vi "Autonomous Independent.vi"() -> ()   [LabVIEW 2015]
doc: "This VI is called when autonomous begins, and will automatically be terminated when autonomous ends. You can carry out timed or sensor driven robot movement independently without needing to return to the caller."
uses:
  <vilib>/Rock Robotics/WPI/Utilities/WPI_GetSetVariantRefNum.vi
  <vilib>/Rock Robotics/Network Tables/NT Read Number.vi
  Robot Global Data.vi
  <vilib>/Rock Robotics/WPI/RobotDrive/WPI_RobotDriveMecanumDrive_Cartesian.vi
  <vilib>/Rock Robotics/Network Tables/NT Write Numeric Array.vi
  <vilib>/Rock Robotics/Network Tables/NT Read Boolean.vi
panel:
  out "Drive Time":dbl
  # "Be sure to right-click and choose Data Operations>>Make Current Value default if you want to save the array values with the VI"
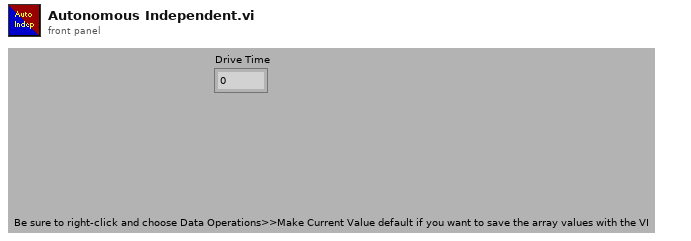
[diagram p1: front panel]
types:
  T1 = typedef "WPI_JoystickDevRef.ctl" = cluster{"Device":T2}
  T2 = typedef "WPI_JoystickDeviceEnum.ctl" = enum16{"USB 0", "USB 1", "USB 2", "USB 3", "USB 4", "USB 5"}
  T3 = typedef "WPI_AccelerometerDevRef.ctl" = cluster{"DevStatus":errorcluster, "Scaling":T4, "Analog Channels":T5, "I2C Bus":T7, "SPI Bus":T8, "Accel Range":T9, "ADXL Axes":T10, "Handle":i32, "Device Address":u8, "Accel Type":enum16{"Analog", "ADXL345 I2C", "ADXL345 SPI", "Internal", "ADXL362 SPI"}}
  T4 = typedef "WPI_AccelerometerScaling.ctl" = cluster{"Gain (VoltsPerG)":dbl, "Center Voltage":dbl}
  T5 = typedef "WPI_AccelerometerAnalogChannels.ctl" = cluster{"X-Axis":T6, "Y-Axis":T6, "Z-Axis":T6}
  T6 = typedef "FPGA_AIChannel.ctl" = enum8{"AI 0", "AI 1", "AI 2", "AI 3", "AI MXP 0", "AI MXP 1", "AI MXP 2", "AI MXP 3", "Invalid"}
  T7 = typedef "i2c_bus.ctl" = enum16{"I2C On-Board", "I2C MXP", "Invalid"}
  T8 = typedef "spi_bus.ctl" = enum16{"SPI On-Board, CS0", "SPI On-Board, CS1", "SPI On-Board, CS2", "SPI On-Board, CS3", "SPI MXP", "Invalid"}
  T9 = typedef "ADXL345 Range.ctl" = u8
  T10 = typedef "WPI_AccelerometerADXL345 Axes.ctl" = cluster{"X-Axis":bool, "Y-Axis":bool, "Z-Axis":bool}
  T11 = typedef "WPI_MotorControlDeviceRef.ctl" = cluster{"DeviceStatus":errorcluster, "Type":T12, "PWM":cluster{"PWM Channel":T13, "DeadBand":T14}, "CAN":cluster{"Device Number":u8, "Control Mode":T15, "Semaphore":T16, "Max Vout":dbl, "TalonSRX Control Mode":T17}, "Invert":bool}
  T12 = typedef "WPI_MotorControlType.ctl" = enum16{"PWM", "CAN", "CANTalonSRX"}
  T13 = typedef "FPGA_DIOPWMChannel.ctl" = enum8{"PWM 0", "PWM 1", "PWM 2", "PWM 3", "PWM 4", "PWM 5", "PWM 6", "PWM 7", "PWM 8", "PWM 9", "PWM MXP 0", "PWM MXP 1", "PWM MXP 2", "PWM MXP 3", "PWM MXP 4", "PWM MXP 5", "PWM MXP 6", "PWM MXP 7", "PWM MXP 8", "PWM MXP 9", "Invalid"}
  T14 = typedef "WPI_PWMDeadband.ctl" = cluster{"Name":string, "maxPositivePwm":i32, "minPositivePwm":i32, "centerPwm":i32, "maxNegativePwm":i32, "minNegativePwm":i32, "angularRange":u16}
  T15 = typedef "WPI_CANJaguar_ControlMode.ctl" = enum8{"Percent VBus", "Current", "Speed", "Position", "Voltage"}
  T16 = typedef "Semaphore RefNum" = refnum<k1>
  T17 = typedef "WPI_CANTalonSRX_APIControlMode.ctl" = enum8{"Percent VBus", "Speed", "Position", "Slave", "Unchanged / Invalid", "Voltage Compensation", "Current", "Motion Profile"}
  T18 = typedef "WPI_RobotDriveDevRef.ctl" = cluster{"DevStatus":errorcluster, "Motors[]":T11[], "Square Inputs":bool, "Max Output":dbl}
  T19 = typedef "eventsource.ctl" = u32
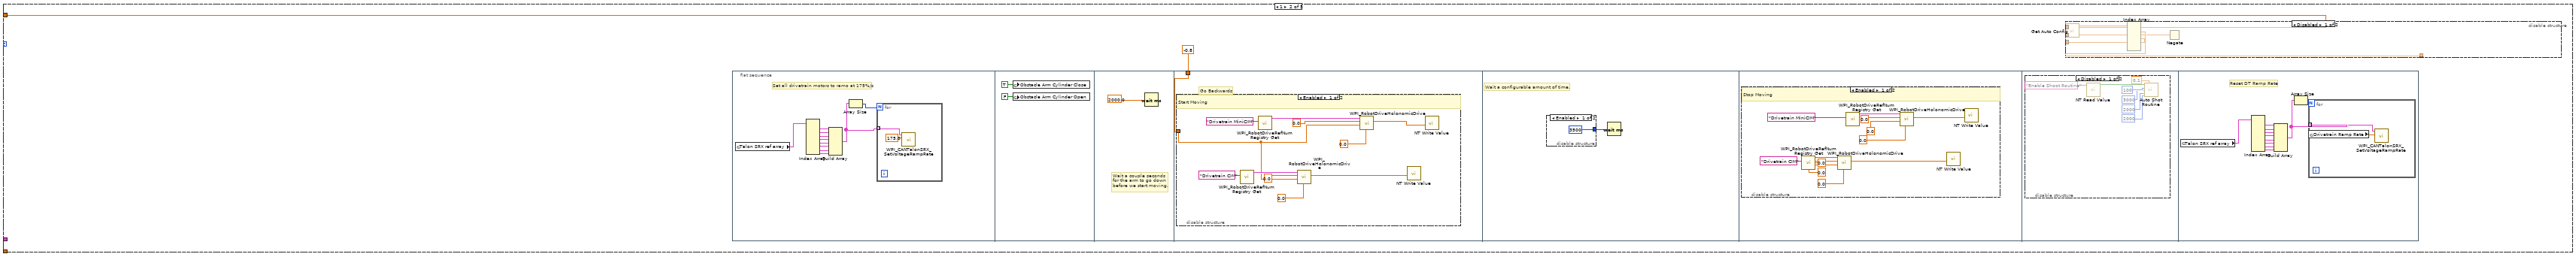
[diagram p3: hidden frame]
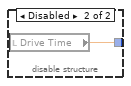
[diagram p6: hidden frame]
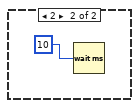
[diagram p14: hidden frame]
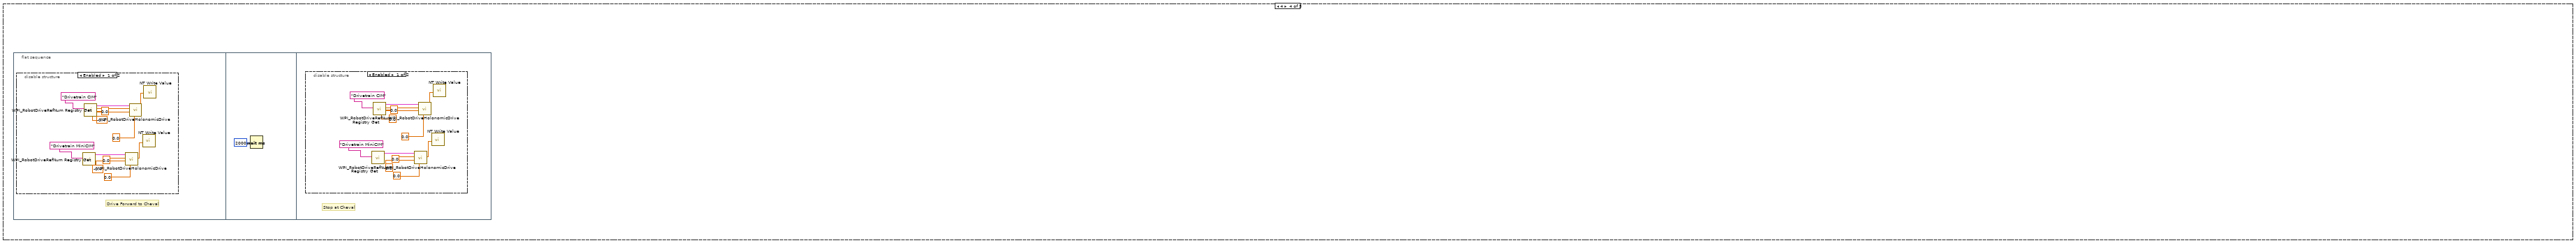
[diagram p19: hidden frame]
diagram:
  (unwired) "This function is run in parallel when the autonomous period begins. It will be terminated automatically when the period ends.\n\nNote that all Driver Station inputs are automatically latched and will not change once auto begins."
  # "Low Bar/Portcullis Auto Routine, with optional shoot routine."
  # "This tells you the autonomous selected\nfrom the dashboard"
  # "Every 20ms, report that we are running autonomous\ncode. Loop will abort the same time as the VI."
  # "This gives you the joystick value\nthat is often the throttle"
  # "This tells you the driver position\nand alliance color"
  n1 = while {
    stop <- FALSE stop-if-true
    n2 = call <vilib>:"WPI_DriverStationReport Robot Code State.vi"("Autonomous"=TRUE) -> ()  [unwired: 10 in, 1 out]
    n3 = Wait (ms)(milliseconds to wait=u32 20) -> ()  [unwired: 1 out]
  }
  n4 = call <vilib>:"WPI_DriverStationGet Alliance Info.vi"() -> ()  [unwired: 12 out]
  n5 = call <vilib>:"WPI_JoystickRefNum Registry Get.vi"("refnum name"="Joystick 0") -> ("JoystickDevRef"=w10:T1)  [unwired: 1 in, 9 out]
  n6 = disable-structure shown="Enabled" {
    disable-tunnel: [w16 _] -> w4
    frame Enabled {
      n7 = call-poly <vilib>:"NT Read Value.vi"("Name"="Drive Time") -> ("Numeric"=w16:dbl)  [unwired: 9 in, 1 out]
    }
    frame Disabled {
    }
  }
  n8 = call <vilib>:"WPI_JoystickGetValues.vi"("JoystickDevRef"=w10) -> ("Axes"=w7:dbl[])  [unwired: 6 in, 4 out]
  n9 = call-poly <vilib>:"NT Read Value.vi"("Name"="Select Autonomous") -> ("Numeric"=w5:dbl)  [unwired: 9 in, 1 out]
  n10 = local write "Drive Time"(w4) -> ()
  n11 = call-poly <vilib>:"NT Write Value.vi"("Numeric Array"=w7, "Name"="Joystick 0/Axes") -> ()  [unwired: 9 in, 1 out]
  n12 = Index Array(array=w7, index=2) -> ()  [unwired: 1 out]
  n13 = flat-sequence {
    tunnel: w5 -> [w20]
    tunnel: [w20] -> w3
    tunnel: [w18] -> w2
    tunnel: [w17] -> w1
    tunnel: w3 -> [w23]
    tunnel: w2 -> [w22]
    tunnel: w1 -> [w21]
    frame #0 {
      # "Initialize Accel."
      n14 = call "2039_GetAccelDeltas.vi"("refnum name"="Internal Accel") -> ("Deltas to apply"=w17:dbl[], "AccelerometerDevRef"=w18:T3)  [unwired: 2 in, 1 out]
    }
    frame #1 {
      n15 = case shown="3" w23 {
        tunnel: w23 -> [_ w25 _ _ _]
        tunnel: w22 -> [_ _ w100 _ _]
        tunnel: w21 -> [_ _ w99 _ _]
        frame 0, Default {
        }
        frame 1 {
          n16 = flat-sequence {
            tunnel: -0.8 -> [w48]
            frame #0 {
              # "Set all drivetrain motors to ramo at 175%/s"
              n17 = global read "Robot Global Data.vi" "Talon SRX ref array"() -> (w42:T11[])
              n18 = Index Array(array=w42) -> (element #1=w35:T11, element #2=w34:T11, element #3=w36:T11, element #4=w37:T11, element #5=w38:T11, element #6=w39:T11, element #7=w40:T11, element #8=w41:T11)  [unwired: 8 in]
              n19 = Build Array(w35, w34, w36, w37, w38, w39, w40, w41) -> (w32:T11[])
              n20 = Array Size(array=w32) -> (size(s)=w33:i32)
              n21 = for {
                N: w33 -> [_]
                tunnel: w32 -> [w44] mode=indexing
                n22 = call <vilib>:"WPI_CANTalonSRX_SetVoltageRampRate.vi"("Throttle Ramp Rate (percent/s)"=175.0, "CAN Talon SRX Ref"=w44) -> ()  [unwired: 8 in, 2 out]
              }
            }
            frame #1 {
              n23 = global write "Robot Global Data.vi" "Obstacle Arm Cylinder Close"(TRUE) -> ()
              n24 = global write "Robot Global Data.vi" "Obstacle Arm Cylinder Open"(FALSE) -> ()
            }
            frame #2 {
              # "Wait a couple seconds\nfor the arm to go down\nbefore we start moving."
              n25 = Wait (ms)(milliseconds to wait=2000.0) -> ()  [unwired: 1 out]
            }
            frame #3 {
              # "Go Backwards"
              n26 = disable-structure shown="Enabled" {
                disable-tunnel: w48 -> [w50 _]
                frame Enabled {
                  # "Start Moving"
                  n27 = call <vilib>:"WPI_RobotDriveRefNum Registry Get.vi"("refnum name"="Drivetrain CIM") -> ("RobotDriveDevRef"=w56:T18)  [unwired: 1 in, 9 out]
                  n28 = call <vilib>:"WPI_RobotDriveRefNum Registry Get.vi"("refnum name"="Drivetrain MiniCIM") -> ("RobotDriveDevRef"=w52:T18)  [unwired: 1 in, 9 out]
                  n29 = call-poly <vilib>:"WPI_RobotDriveHolonomicDrive.vi"("Rotation"=0.0, "Y"=w50, "X"=0.0 ("X axis value"), "RobotDriveDevRef"=w56) -> ("Motor Values"=w57:dbl[])  [unwired: 5 in, 2 out]
                  n30 = call-poly <vilib>:"WPI_RobotDriveHolonomicDrive.vi"("Rotation"=0.0, "Y"=w50, "X"=0.0 ("X axis value"), "RobotDriveDevRef"=w52) -> ("Motor Values"=w54:dbl[])  [unwired: 5 in, 2 out]
                  n31 = call-poly <vilib>:"NT Write Value.vi"("Numeric Array"=w57) -> ()  [unwired: 10 in, 1 out]
                  n32 = call-poly <vilib>:"NT Write Value.vi"("Numeric Array"=w54) -> ()  [unwired: 10 in, 1 out]
                }
                frame Disabled {
                }
              }
            }
            frame #4 {
              # "Wait a configurable amount of time."
              n33 = disable-structure shown="Enabled" {
                disable-tunnel: [u32 3500 ("milliseconds to wait") w62] -> w60
                frame Enabled {
                }
                frame Disabled {
                  n34 = local read "Drive Time"() -> (w62:dbl)
                }
              }
              n35 = Wait (ms)(milliseconds to wait=w60) -> ()  [unwired: 1 out]
            }
            frame #5 {
              n36 = disable-structure shown="Enabled" {
                frame Enabled {
                  # "Stop Moving"
                  n37 = call <vilib>:"WPI_RobotDriveRefNum Registry Get.vi"("refnum name"="Drivetrain CIM") -> ("RobotDriveDevRef"=w70:T18)  [unwired: 1 in, 9 out]
                  n38 = call-poly <vilib>:"WPI_RobotDriveHolonomicDrive.vi"("Rotation"=0.0, "Y"=0.0 ("X axis value"), "X"=0.0 ("X axis value"), "RobotDriveDevRef"=w70) -> ("Motor Values"=w71:dbl[])  [unwired: 5 in, 2 out]
                  n39 = call <vilib>:"WPI_RobotDriveRefNum Registry Get.vi"("refnum name"="Drivetrain MiniCIM") -> ("RobotDriveDevRef"=w64:T18)  [unwired: 1 in, 9 out]
                  n40 = call-poly <vilib>:"WPI_RobotDriveHolonomicDrive.vi"("Rotation"=0.0, "Y"=0.0 ("X axis value"), "X"=0.0 ("X axis value"), "RobotDriveDevRef"=w64) -> ("Motor Values"=w66:dbl[])  [unwired: 5 in, 2 out]
                  n41 = call-poly <vilib>:"NT Write Value.vi"("Numeric Array"=w71) -> ()  [unwired: 10 in, 1 out]
                  n42 = call-poly <vilib>:"NT Write Value.vi"("Numeric Array"=w66) -> ()  [unwired: 10 in, 1 out]
                }
                frame Disabled {
                }
              }
            }
            frame #6 {
              n43 = disable-structure shown="Disabled" {
                frame Disabled {
                  n44 = call-poly <vilib>:"NT Read Value.vi"("Name"="Enable Shoot Routine") -> ("Boolean"=w80:bool)  [unwired: 9 in, 1 out]
                  n45 = call "Auto Shot Routine.vi"("Enable"=w80, "Speed to run intake motor (negated)"=0.1, "Time to wait after boulder out"=100, 7:3000, "Wait for SpinUp"=2000, "Wait for Shot Time"=2000) -> ()  [unwired: 10 in]
                }
                frame Enabled {
                }
              }
            }
            frame #7 {
              # "Reset DT Ramp Rate"
              n46 = global read "Robot Global Data.vi" "Talon SRX ref array"() -> (w92:T11[])
              n47 = Index Array(array=w92) -> (element #1=w85:T11, element #2=w84:T11, element #3=w86:T11, element #4=w87:T11, element #5=w88:T11, element #6=w89:T11, element #7=w90:T11, element #8=w91:T11)  [unwired: 8 in]
              n48 = Build Array(w85, w84, w86, w87, w88, w89, w90, w91) -> (w82:T11[])
              n49 = Array Size(array=w82) -> (size(s)=w83:i32)
              n50 = for {
                N: w83 -> [_]
                tunnel: w82 -> [w94] mode=indexing
                n51 = global read "Robot Global Data.vi" "Drivetrain Ramp Rate"() -> (w93:dbl)
                n52 = call <vilib>:"WPI_CANTalonSRX_SetVoltageRampRate.vi"("Throttle Ramp Rate (percent/s)"=w93, "CAN Talon SRX Ref"=w94) -> ()  [unwired: 8 in, 2 out]
              }
            }
          }
          n53 = disable-structure shown="Disabled" {
            disable-tunnel: w25 -> [w30 _]
            disable-tunnel: [w29 _] -> _
            disable-tunnel: [w27 _] -> _
            disable-tunnel: [w26 _] -> _
            frame Disabled {
              n54 = call "Get Auto Config.vi"("Numeric"=w30) -> ("Numeric Array"=w31:dbl[])  [unwired: 10 in]
              n55 = Index Array(array=w31) -> (element #1=w29:dbl, element #2=w28:dbl, element #3=w26:dbl)  [unwired: 6 in, 3 out]
              n56 = Negate(x=w28) -> (-x=w27:dbl)
            }
            frame Enabled {
            }
          }
        }
        frame 2 {
          # "Hopefully this will run in parallel"
          # "Can be written as needed..."
          n57 = flat-sequence {
            tunnel: w97 -> [w113]
            tunnel: [w111] -> _
            tunnel: [w111] -> w96
            tunnel: w96 -> [w116]
            tunnel: [w116] -> w95
            tunnel: w95 -> [w125]
            frame #0 {
              n58 = disable-structure shown="Enabled" {
                frame Enabled {
                  w101 = 0.0
                  w102 = 0.0 ("X axis value")
                  # "Start Moving"
                  n59 = call <vilib>:"WPI_RobotDriveRefNum Registry Get.vi"("refnum name"="Drivetrain CIM") -> ("RobotDriveDevRef"=w108:T18)  [unwired: 1 in, 9 out]
                  n60 = call <vilib>:"WPI_RobotDriveRefNum Registry Get.vi"("refnum name"="Drivetrain MiniCIM") -> ("RobotDriveDevRef"=w105:T18)  [unwired: 1 in, 9 out]
                  n61 = call-poly <vilib>:"WPI_RobotDriveHolonomicDrive.vi"("Rotation"=w102, "Y"=-0.8 ("X axis value"), "X"=w102, "RobotDriveDevRef"=w105) -> ("Motor Values"=w107:dbl[])  [unwired: 5 in, 2 out]
                  n62 = call-poly <vilib>:"WPI_RobotDriveHolonomicDrive.vi"("Rotation"=w101, "Y"=-0.8, "X"=w101, "RobotDriveDevRef"=w108) -> ("Motor Values"=w109:dbl[])  [unwired: 5 in, 2 out]
                  n63 = call-poly <vilib>:"NT Write Value.vi"("Numeric Array"=w109) -> ()  [unwired: 10 in, 1 out]
                  n64 = call-poly <vilib>:"NT Write Value.vi"("Numeric Array"=w107) -> ()  [unwired: 10 in, 1 out]
                }
                frame Disabled {
                }
              }
            }
            frame #1 {
              n65 = event shown="[0] <Acceleration Spike Event>: User Event;  Timeout" {
                selector: w113 -> [_]
                dyn-events: _ -> [_]
                timeout: 2500 -> [_]
                tunnel: [w114] -> w111
                event User Event; Timeout {
                  # "Wait until either Timeout or accel change."
                  n66 = event-data() -> ("Source"=w114:T19)  [unwired: 1 in, 2 out]
                  n67 = Wait (ms)(milliseconds to wait=10) -> ()  [unwired: 1 out]
                }
              }
            }
            frame #2 {
              n68 = disable-structure shown="Enabled" {
                frame Enabled {
                  w117 = 0.0
                  w118 = 0.0 ("X axis value")
                  # "Stop Moving"
                  n69 = call <vilib>:"WPI_RobotDriveRefNum Registry Get.vi"("refnum name"="Drivetrain CIM") -> ("RobotDriveDevRef"=w122:T18)  [unwired: 1 in, 9 out]
                  n70 = call <vilib>:"WPI_RobotDriveRefNum Registry Get.vi"("refnum name"="Drivetrain MiniCIM") -> ("RobotDriveDevRef"=w119:T18)  [unwired: 1 in, 9 out]
                  n71 = call-poly <vilib>:"WPI_RobotDriveHolonomicDrive.vi"("Rotation"=w117, "Y"=w117, "X"=w117, "RobotDriveDevRef"=w122) -> ("Motor Values"=w123:dbl[])  [unwired: 5 in, 2 out]
                  n72 = call-poly <vilib>:"WPI_RobotDriveHolonomicDrive.vi"("Rotation"=w118, "Y"=w118, "X"=w118, "RobotDriveDevRef"=w119) -> ("Motor Values"=w121:dbl[])  [unwired: 5 in, 2 out]
                  n73 = call-poly <vilib>:"NT Write Value.vi"("Numeric Array"=w123) -> ()  [unwired: 10 in, 1 out]
                  n74 = call-poly <vilib>:"NT Write Value.vi"("Numeric Array"=w121) -> ()  [unwired: 10 in, 1 out]
                }
                frame Disabled {
                }
              }
            }
            frame #3 {
              n75 = case shown="1, Default" w125 {
                frame 1, Default {
                  # "Back up a smidge if we timed out"
                  n76 = flat-sequence {
                    frame #0 {
                      n77 = disable-structure shown="Enabled" {
                        frame Enabled {
                          n78 = call <vilib>:"WPI_RobotDriveRefNum Registry Get.vi"("refnum name"="Drivetrain CIM") -> ("RobotDriveDevRef"=w133:T18)  [unwired: 1 in, 9 out]
                          n79 = call <vilib>:"WPI_RobotDriveRefNum Registry Get.vi"("refnum name"="Drivetrain MiniCIM") -> ("RobotDriveDevRef"=w127:T18)  [unwired: 1 in, 9 out]
                          n80 = call-poly <vilib>:"WPI_RobotDriveHolonomicDrive.vi"("Rotation"=0.0, "Y"=0.0 ("X axis value"), "X"=0.5 ("X axis value"), "RobotDriveDevRef"=w127) -> ("Motor Values"=w128:dbl[])  [unwired: 5 in, 2 out]
                          n81 = call-poly <vilib>:"WPI_RobotDriveHolonomicDrive.vi"("Rotation"=0.0, "Y"=0.5 ("X axis value"), "X"=0.0 ("X axis value"), "RobotDriveDevRef"=w133) -> ("Motor Values"=w134:dbl[])  [unwired: 5 in, 2 out]
                          n82 = call-poly <vilib>:"NT Write Value.vi"("Numeric Array"=w128) -> ()  [unwired: 10 in, 1 out]
                          n83 = call-poly <vilib>:"NT Write Value.vi"("Numeric Array"=w134) -> ()  [unwired: 10 in, 1 out]
                        }
                        frame Disabled {
                        }
                      }
                    }
                    frame #1 {
                      n84 = Wait (ms)(milliseconds to wait=300) -> ()  [unwired: 1 out]
                    }
                    frame #2 {
                      n85 = disable-structure shown="Enabled" {
                        frame Enabled {
                          n86 = call <vilib>:"WPI_RobotDriveRefNum Registry Get.vi"("refnum name"="Drivetrain CIM") -> ("RobotDriveDevRef"=w146:T18)  [unwired: 1 in, 9 out]
                          n87 = call <vilib>:"WPI_RobotDriveRefNum Registry Get.vi"("refnum name"="Drivetrain MiniCIM") -> ("RobotDriveDevRef"=w140:T18)  [unwired: 1 in, 9 out]
                          n88 = call-poly <vilib>:"WPI_RobotDriveHolonomicDrive.vi"("Rotation"=0.0, "Y"=0.0 ("X axis value"), "X"=0.0 ("X axis value"), "RobotDriveDevRef"=w140) -> ("Motor Values"=w141:dbl[])  [unwired: 5 in, 2 out]
                          n89 = call-poly <vilib>:"WPI_RobotDriveHolonomicDrive.vi"("Rotation"=0.0, "Y"=0.0 ("X axis value"), "X"=0.0 ("X axis value"), "RobotDriveDevRef"=w146) -> ("Motor Values"=w147:dbl[])  [unwired: 5 in, 2 out]
                          n90 = call-poly <vilib>:"NT Write Value.vi"("Numeric Array"=w141) -> ()  [unwired: 10 in, 1 out]
                          n91 = call-poly <vilib>:"NT Write Value.vi"("Numeric Array"=w147) -> ()  [unwired: 10 in, 1 out]
                        }
                        frame Disabled {
                        }
                      }
                    }
                  }
                }
                frame 2 {
                  n92 = Wait (ms)(milliseconds to wait=10) -> ()  [unwired: 1 out]
                }
              }
            }
            frame #4 {
              n93 = global write "Robot Global Data.vi" "Obstacle Arm Cylinder Close"(TRUE) -> ()
              n94 = global write "Robot Global Data.vi" "Obstacle Arm Cylinder Open"(FALSE) -> ()
            }
            frame #5 {
              n95 = Wait (ms)(milliseconds to wait=2000) -> ()  [unwired: 1 out]
            }
            frame #6 {
              # "Go forth and conquer, o brave one."
              n96 = flat-sequence {
                frame #0 {
                  n97 = disable-structure shown="Enabled" {
                    frame Enabled {
                      n98 = call <vilib>:"WPI_RobotDriveRefNum Registry Get.vi"("refnum name"="Drivetrain CIM") -> ("RobotDriveDevRef"=w162:T18)  [unwired: 1 in, 9 out]
                      n99 = call <vilib>:"WPI_RobotDriveRefNum Registry Get.vi"("refnum name"="Drivetrain MiniCIM") -> ("RobotDriveDevRef"=w156:T18)  [unwired: 1 in, 9 out]
                      n100 = call-poly <vilib>:"WPI_RobotDriveHolonomicDrive.vi"("Rotation"=0.0, "Y"=0.0 ("X axis value"), "X"=-1.0 ("X axis value"), "RobotDriveDevRef"=w156) -> ("Motor Values"=w157:dbl[])  [unwired: 5 in, 2 out]
                      n101 = call-poly <vilib>:"WPI_RobotDriveHolonomicDrive.vi"("Rotation"=0.0, "Y"=-1.0 ("X axis value"), "X"=0.0 ("X axis value"), "RobotDriveDevRef"=w162) -> ("Motor Values"=w163:dbl[])  [unwired: 5 in, 2 out]
                      n102 = call-poly <vilib>:"NT Write Value.vi"("Numeric Array"=w157) -> ()  [unwired: 10 in, 1 out]
                      n103 = call-poly <vilib>:"NT Write Value.vi"("Numeric Array"=w163) -> ()  [unwired: 10 in, 1 out]
                    }
                    frame Disabled {
                    }
                  }
                }
                frame #1 {
                  n104 = Wait (ms)(milliseconds to wait=3500) -> ()  [unwired: 1 out]
                }
                frame #2 {
                  n105 = disable-structure shown="Enabled" {
                    frame Enabled {
                      n106 = call <vilib>:"WPI_RobotDriveRefNum Registry Get.vi"("refnum name"="Drivetrain CIM") -> ("RobotDriveDevRef"=w175:T18)  [unwired: 1 in, 9 out]
                      n107 = call <vilib>:"WPI_RobotDriveRefNum Registry Get.vi"("refnum name"="Drivetrain MiniCIM") -> ("RobotDriveDevRef"=w169:T18)  [unwired: 1 in, 9 out]
                      n108 = call-poly <vilib>:"WPI_RobotDriveHolonomicDrive.vi"("Rotation"=0.0, "Y"=0.0 ("X axis value"), "X"=0.0 ("X axis value"), "RobotDriveDevRef"=w169) -> ("Motor Values"=w170:dbl[])  [unwired: 5 in, 2 out]
                      n109 = call-poly <vilib>:"WPI_RobotDriveHolonomicDrive.vi"("Rotation"=0.0, "Y"=0.0 ("X axis value"), "X"=0.0 ("X axis value"), "RobotDriveDevRef"=w175) -> ("Motor Values"=w176:dbl[])  [unwired: 5 in, 2 out]
                      n110 = call-poly <vilib>:"NT Write Value.vi"("Numeric Array"=w170) -> ()  [unwired: 10 in, 1 out]
                      n111 = call-poly <vilib>:"NT Write Value.vi"("Numeric Array"=w176) -> ()  [unwired: 10 in, 1 out]
                    }
                    frame Disabled {
                    }
                  }
                }
              }
            }
          }
          n112 = call "2039_AccelSpike.vi"("Threshold"=1.0, "Delta Array"=w99, "AccelerometerDevRef"=w100) -> ("Event Registration Refnum"=w97:refnum<event-registration>)  [unwired: 7 in, 1 out]
          n113 = flat-sequence {
            frame #0 {
              n114 = disable-structure shown="Enabled" {
                frame Enabled {
                  n115 = call <vilib>:"WPI_RobotDriveRefNum Registry Get.vi"("refnum name"="Drivetrain MiniCIM") -> ("RobotDriveDevRef"=w181:T18)  [unwired: 1 in, 9 out]
                  n116 = call <vilib>:"WPI_RobotDriveRefNum Registry Get.vi"("refnum name"="Drivetrain CIM") -> ("RobotDriveDevRef"=w187:T18)  [unwired: 1 in, 9 out]
                  n117 = call-poly <vilib>:"WPI_RobotDriveHolonomicDrive.vi"("Rotation"=0.0, "Y"=0.6 ("X axis value"), "X"=0.0 ("X axis value"), "RobotDriveDevRef"=w181) -> ("Motor Values"=w182:dbl[])  [unwired: 5 in, 2 out]
                  n118 = call-poly <vilib>:"WPI_RobotDriveHolonomicDrive.vi"("Rotation"=0.0, "Y"=0.6 ("X axis value"), "X"=0.0 ("X axis value"), "RobotDriveDevRef"=w187) -> ("Motor Values"=w188:dbl[])  [unwired: 5 in, 2 out]
                  n119 = call-poly <vilib>:"NT Write Value.vi"("Numeric Array"=w182) -> ()  [unwired: 10 in, 1 out]
                  n120 = call-poly <vilib>:"NT Write Value.vi"("Numeric Array"=w188) -> ()  [unwired: 10 in, 1 out]
                }
                frame Disabled {
                }
              }
            }
            frame #1 {
              n121 = Wait (ms)(milliseconds to wait=u32 2500) -> ()  [unwired: 1 out]
            }
            frame #2 {
              n122 = disable-structure shown="Enabled" {
                frame Enabled {
                  n123 = call <vilib>:"WPI_RobotDriveRefNum Registry Get.vi"("refnum name"="Drivetrain MiniCIM") -> ("RobotDriveDevRef"=w194:T18)  [unwired: 1 in, 9 out]
                  n124 = call <vilib>:"WPI_RobotDriveRefNum Registry Get.vi"("refnum name"="Drivetrain CIM") -> ("RobotDriveDevRef"=w200:T18)  [unwired: 1 in, 9 out]
                  n125 = call-poly <vilib>:"WPI_RobotDriveHolonomicDrive.vi"("Rotation"=0.3, "Y"=0.0 ("X axis value"), "X"=0.0 ("X axis value"), "RobotDriveDevRef"=w194) -> ("Motor Values"=w195:dbl[])  [unwired: 5 in, 2 out]
                  n126 = call-poly <vilib>:"WPI_RobotDriveHolonomicDrive.vi"("Rotation"=0.3, "Y"=0.0 ("X axis value"), "X"=0.0 ("X axis value"), "RobotDriveDevRef"=w200) -> ("Motor Values"=w201:dbl[])  [unwired: 5 in, 2 out]
                  n127 = call-poly <vilib>:"NT Write Value.vi"("Numeric Array"=w195) -> ()  [unwired: 10 in, 1 out]
                  n128 = call-poly <vilib>:"NT Write Value.vi"("Numeric Array"=w201) -> ()  [unwired: 10 in, 1 out]
                }
                frame Disabled {
                }
              }
            }
            frame #3 {
              n129 = Wait (ms)(milliseconds to wait=u32 650) -> ()  [unwired: 1 out]
            }
            frame #4 {
              n130 = global write "Robot Global Data.vi" "Center"(TRUE) -> ()
            }
            frame #5 {
              n131 = Wait (ms)(milliseconds to wait=u32 1200) -> ()  [unwired: 1 out]
            }
            frame #6 {
              n132 = call <vilib>:"WPI_MotorControlRefNum Registry Get.vi"("refnum name"="Pickup Motor") -> ("error out"=w215:errorcluster, "MotorControlDevRef"=w214:T11)  [unwired: 9 in]
              n133 = call "2039_BackTalonOut.vi"("Throttle Ramp Rate (percent/s)"=1000.0, "Invert Stop Condition"=TRUE, "Speed to run motor (will be negated)"=0.05, "error in (no error)"=w215, "DIO Ref Name"="Shoot Photoeye", "Brake"=TRUE, "CAN Talon SRX Ref"=w214) -> ()  [unwired: 3 in, 2 out]
            }
            frame #7 {
              n134 = global write "Robot Global Data.vi" "Center"(FALSE) -> ()
              n135 = global write "Robot Global Data.vi" "Shot Prep"(TRUE) -> ()
              n136 = global write "Robot Global Data.vi" "High Shot Speed"(FALSE) -> ()
              n137 = global write "Robot Global Data.vi" "Pickup"(TRUE) -> ()
            }
            frame #8 {
              n138 = Wait (ms)(milliseconds to wait=u32 3000) -> ()  [unwired: 1 out]
            }
            frame #9 {
              n139 = global write "Robot Global Data.vi" "Shot Prep"(FALSE) -> ()
              n140 = global write "Robot Global Data.vi" "Pickup"(FALSE) -> ()
            }
          }
        }
        frame 4 {
          # "Love Tap Outer Works"
          n141 = flat-sequence {
            frame #0 {
              # "Drive Forward to Cheval"
              n142 = disable-structure shown="Enabled" {
                frame Enabled {
                  n143 = call <vilib>:"WPI_RobotDriveRefNum Registry Get.vi"("refnum name"="Drivetrain MiniCIM") -> ("RobotDriveDevRef"=w224:T18)  [unwired: 1 in, 9 out]
                  n144 = call <vilib>:"WPI_RobotDriveRefNum Registry Get.vi"("refnum name"="Drivetrain CIM") -> ("RobotDriveDevRef"=w230:T18)  [unwired: 1 in, 9 out]
                  n145 = call-poly <vilib>:"WPI_RobotDriveHolonomicDrive.vi"("Rotation"=0.0, "Y"=-0.4 ("X axis value"), "X"=0.0 ("X axis value"), "RobotDriveDevRef"=w224) -> ("Motor Values"=w225:dbl[])  [unwired: 5 in, 2 out]
                  n146 = call-poly <vilib>:"WPI_RobotDriveHolonomicDrive.vi"("Rotation"=0.0, "Y"=-0.4 ("X axis value"), "X"=0.0 ("X axis value"), "RobotDriveDevRef"=w230) -> ("Motor Values"=w231:dbl[])  [unwired: 5 in, 2 out]
                  n147 = call-poly <vilib>:"NT Write Value.vi"("Numeric Array"=w225) -> ()  [unwired: 10 in, 1 out]
                  n148 = call-poly <vilib>:"NT Write Value.vi"("Numeric Array"=w231) -> ()  [unwired: 10 in, 1 out]
                }
                frame Disabled {
                }
              }
            }
            frame #1 {
              n149 = Wait (ms)(milliseconds to wait=u32 2000) -> ()  [unwired: 1 out]
            }
            frame #2 {
              # "Stop at Cheval"
              n150 = disable-structure shown="Enabled" {
                frame Enabled {
                  n151 = call <vilib>:"WPI_RobotDriveRefNum Registry Get.vi"("refnum name"="Drivetrain MiniCIM") -> ("RobotDriveDevRef"=w237:T18)  [unwired: 1 in, 9 out]
                  n152 = call <vilib>:"WPI_RobotDriveRefNum Registry Get.vi"("refnum name"="Drivetrain CIM") -> ("RobotDriveDevRef"=w243:T18)  [unwired: 1 in, 9 out]
                  n153 = call-poly <vilib>:"WPI_RobotDriveHolonomicDrive.vi"("Rotation"=0.0, "Y"=0.0 ("X axis value"), "X"=0.0 ("X axis value"), "RobotDriveDevRef"=w237) -> ("Motor Values"=w238:dbl[])  [unwired: 5 in, 2 out]
                  n154 = call-poly <vilib>:"WPI_RobotDriveHolonomicDrive.vi"("Rotation"=0.0, "Y"=0.0 ("X axis value"), "X"=0.0 ("X axis value"), "RobotDriveDevRef"=w243) -> ("Motor Values"=w244:dbl[])  [unwired: 5 in, 2 out]
                  n155 = call-poly <vilib>:"NT Write Value.vi"("Numeric Array"=w238) -> ()  [unwired: 10 in, 1 out]
                  n156 = call-poly <vilib>:"NT Write Value.vi"("Numeric Array"=w244) -> ()  [unwired: 10 in, 1 out]
                }
                frame Disabled {
                }
              }
            }
          }
          n157 = flat-sequence {
            frame #0 {
              n158 = disable-structure shown="Enabled" {
                frame Enabled {
                  # "Moves forward for 5 sec"
                  n159 = call <vilib>:"WPI_RobotDriveRefNum Registry Get.vi"("refnum name"="Drivetrain CIM") -> ("RobotDriveDevRef"=w255:T18)  [unwired: 1 in, 9 out]
                  n160 = call <vilib>:"WPI_RobotDriveRefNum Registry Get.vi"("refnum name"="Drivetrain MiniCIM") -> ("RobotDriveDevRef"=w249:T18)  [unwired: 1 in, 9 out]
                  n161 = call-poly <vilib>:"WPI_RobotDriveHolonomicDrive.vi"("Rotation"=0.0, "Y"=-0.4 ("X axis value"), "X"=0.0 ("X axis value"), "RobotDriveDevRef"=w255) -> ("Motor Values"=w256:dbl[])  [unwired: 5 in, 2 out]
                  n162 = call-poly <vilib>:"WPI_RobotDriveHolonomicDrive.vi"("Rotation"=0.0, "Y"=-0.4 ("X axis value"), "X"=0.0 ("X axis value"), "RobotDriveDevRef"=w249) -> ("Motor Values"=w251:dbl[])  [unwired: 5 in, 2 out]
                  n163 = call-poly <vilib>:"NT Write Value.vi"("Numeric Array"=w256) -> ()  [unwired: 10 in, 1 out]
                  n164 = call-poly <vilib>:"NT Write Value.vi"("Numeric Array"=w251) -> ()  [unwired: 10 in, 1 out]
                }
                frame Disabled {
                }
              }
            }
            frame #1 {
              n165 = Wait (ms)(milliseconds to wait=u32 2000) -> ()  [unwired: 1 out]
            }
            frame #2 {
              n166 = call <vilib>:"WPI_RobotDriveRefNum Registry Get.vi"("refnum name"="Drivetrain CIM") -> ("RobotDriveDevRef"=w268:T18)  [unwired: 1 in, 9 out]
              n167 = call <vilib>:"WPI_RobotDriveRefNum Registry Get.vi"("refnum name"="Drivetrain MiniCIM") -> ("RobotDriveDevRef"=w262:T18)  [unwired: 1 in, 9 out]
              n168 = call-poly <vilib>:"WPI_RobotDriveHolonomicDrive.vi"("Rotation"=0.0, "Y"=0.0 ("X axis value"), "X"=0.0 ("X axis value"), "RobotDriveDevRef"=w268) -> ("Motor Values"=w269:dbl[])  [unwired: 5 in, 2 out]
              n169 = call-poly <vilib>:"NT Write Value.vi"("Numeric Array"=w269) -> ()  [unwired: 10 in, 1 out]
              n170 = call-poly <vilib>:"WPI_RobotDriveHolonomicDrive.vi"("Rotation"=0.0, "Y"=0.0 ("X axis value"), "X"=0.0 ("X axis value"), "RobotDriveDevRef"=w262) -> ("Motor Values"=w264:dbl[])  [unwired: 5 in, 2 out]
              n171 = call-poly <vilib>:"NT Write Value.vi"("Numeric Array"=w264) -> ()  [unwired: 10 in, 1 out]
            }
          }
        }
        frame 3 {
          # "Cheval de Frise"
          # "The idea of this diagram is to start as close to the low-bar as possible, strafing over the the obstacale, then drive forward over the object. one on the \"other side,\" we move into a position to fire."
          n172 = flat-sequence {
            frame #0 {
              # "Drive Forward to Cheval"
              n173 = disable-structure shown="Enabled" {
                frame Enabled {
                  n174 = call <vilib>:"WPI_RobotDriveRefNum Registry Get.vi"("refnum name"="Drivetrain MiniCIM") -> ("RobotDriveDevRef"=w274:T18)  [unwired: 1 in, 9 out]
                  n175 = call <vilib>:"WPI_RobotDriveRefNum Registry Get.vi"("refnum name"="Drivetrain CIM") -> ("RobotDriveDevRef"=w280:T18)  [unwired: 1 in, 9 out]
                  n176 = call-poly <vilib>:"WPI_RobotDriveHolonomicDrive.vi"("Rotation"=0.0, "Y"=-0.4 ("X axis value"), "X"=0.0 ("X axis value"), "RobotDriveDevRef"=w274) -> ("Motor Values"=w275:dbl[])  [unwired: 5 in, 2 out]
                  n177 = call-poly <vilib>:"WPI_RobotDriveHolonomicDrive.vi"("Rotation"=0.0, "Y"=-0.4 ("X axis value"), "X"=0.0 ("X axis value"), "RobotDriveDevRef"=w280) -> ("Motor Values"=w281:dbl[])  [unwired: 5 in, 2 out]
                  n178 = call-poly <vilib>:"NT Write Value.vi"("Numeric Array"=w275) -> ()  [unwired: 10 in, 1 out]
                  n179 = call-poly <vilib>:"NT Write Value.vi"("Numeric Array"=w281) -> ()  [unwired: 10 in, 1 out]
                }
                frame Disabled {
                }
              }
            }
            frame #1 {
              n180 = Wait (ms)(milliseconds to wait=u32 2000) -> ()  [unwired: 1 out]
            }
            frame #2 {
              # "Stop at Cheval"
              n181 = disable-structure shown="Enabled" {
                frame Enabled {
                  n182 = call <vilib>:"WPI_RobotDriveRefNum Registry Get.vi"("refnum name"="Drivetrain MiniCIM") -> ("RobotDriveDevRef"=w287:T18)  [unwired: 1 in, 9 out]
                  n183 = call <vilib>:"WPI_RobotDriveRefNum Registry Get.vi"("refnum name"="Drivetrain CIM") -> ("RobotDriveDevRef"=w293:T18)  [unwired: 1 in, 9 out]
                  n184 = call-poly <vilib>:"WPI_RobotDriveHolonomicDrive.vi"("Rotation"=0.0, "Y"=0.0 ("X axis value"), "X"=0.0 ("X axis value"), "RobotDriveDevRef"=w287) -> ("Motor Values"=w288:dbl[])  [unwired: 5 in, 2 out]
                  n185 = call-poly <vilib>:"WPI_RobotDriveHolonomicDrive.vi"("Rotation"=0.0, "Y"=0.0 ("X axis value"), "X"=0.0 ("X axis value"), "RobotDriveDevRef"=w293) -> ("Motor Values"=w294:dbl[])  [unwired: 5 in, 2 out]
                  n186 = call-poly <vilib>:"NT Write Value.vi"("Numeric Array"=w288) -> ()  [unwired: 10 in, 1 out]
                  n187 = call-poly <vilib>:"NT Write Value.vi"("Numeric Array"=w294) -> ()  [unwired: 10 in, 1 out]
                }
                frame Disabled {
                }
              }
            }
            frame #3 {
              n188 = Wait (ms)(milliseconds to wait=u32 500) -> ()  [unwired: 1 out]
            }
            frame #4 {
              # "Back up a smidge"
              n189 = disable-structure shown="Disabled" {
                frame Disabled {
                  n190 = call <vilib>:"WPI_RobotDriveRefNum Registry Get.vi"("refnum name"="Drivetrain CIM") -> ("RobotDriveDevRef"=w306:T18)  [unwired: 1 in, 9 out]
                  n191 = call <vilib>:"WPI_RobotDriveRefNum Registry Get.vi"("refnum name"="Drivetrain MiniCIM") -> ("RobotDriveDevRef"=w300:T18)  [unwired: 1 in, 9 out]
                  n192 = call-poly <vilib>:"WPI_RobotDriveHolonomicDrive.vi"("Rotation"=0.0, "Y"=0.0 ("X axis value"), "X"=0.5 ("X axis value"), "RobotDriveDevRef"=w300) -> ("Motor Values"=w301:dbl[])  [unwired: 5 in, 2 out]
                  n193 = call-poly <vilib>:"WPI_RobotDriveHolonomicDrive.vi"("Rotation"=0.0, "Y"=0.5 ("X axis value"), "X"=0.0 ("X axis value"), "RobotDriveDevRef"=w306) -> ("Motor Values"=w307:dbl[])  [unwired: 5 in, 2 out]
                  n194 = call-poly <vilib>:"NT Write Value.vi"("Numeric Array"=w301) -> ()  [unwired: 10 in, 1 out]
                  n195 = call-poly <vilib>:"NT Write Value.vi"("Numeric Array"=w307) -> ()  [unwired: 10 in, 1 out]
                }
                frame Enabled {
                }
              }
            }
            frame #5 {
              n196 = Wait (ms)(milliseconds to wait=u32 200) -> ()  [unwired: 1 out]
            }
            frame #6 {
              # "Stop again"
              n197 = disable-structure shown="Enabled" {
                frame Enabled {
                  n198 = call <vilib>:"WPI_RobotDriveRefNum Registry Get.vi"("refnum name"="Drivetrain CIM") -> ("RobotDriveDevRef"=w319:T18)  [unwired: 1 in, 9 out]
                  n199 = call <vilib>:"WPI_RobotDriveRefNum Registry Get.vi"("refnum name"="Drivetrain MiniCIM") -> ("RobotDriveDevRef"=w313:T18)  [unwired: 1 in, 9 out]
                  n200 = call-poly <vilib>:"WPI_RobotDriveHolonomicDrive.vi"("Rotation"=0.0, "Y"=0.0 ("X axis value"), "X"=0.0 ("X axis value"), "RobotDriveDevRef"=w313) -> ("Motor Values"=w314:dbl[])  [unwired: 5 in, 2 out]
                  n201 = call-poly <vilib>:"WPI_RobotDriveHolonomicDrive.vi"("Rotation"=0.0, "Y"=0.0 ("X axis value"), "X"=0.0 ("X axis value"), "RobotDriveDevRef"=w319) -> ("Motor Values"=w320:dbl[])  [unwired: 5 in, 2 out]
                  n202 = call-poly <vilib>:"NT Write Value.vi"("Numeric Array"=w314) -> ()  [unwired: 10 in, 1 out]
                  n203 = call-poly <vilib>:"NT Write Value.vi"("Numeric Array"=w320) -> ()  [unwired: 10 in, 1 out]
                }
                frame Disabled {
                }
              }
            }
            frame #7 {
              n204 = Wait (ms)(milliseconds to wait=u32 1000) -> ()  [unwired: 1 out]
            }
            frame #8 {
              n205 = global write "Robot Global Data.vi" "Obstacle Arm Cylinder Close"(TRUE) -> ()
              n206 = global write "Robot Global Data.vi" "Obstacle Arm Cylinder Open"(FALSE) -> ()
            }
            frame #9 {
              n207 = Wait (ms)(milliseconds to wait=u32 2000) -> ()  [unwired: 1 out]
            }
            frame #10 {
              n208 = disable-structure shown="Enabled" {
                frame Enabled {
                  n209 = call <vilib>:"WPI_RobotDriveRefNum Registry Get.vi"("refnum name"="Drivetrain MiniCIM") -> ("RobotDriveDevRef"=w329:T18)  [unwired: 1 in, 9 out]
                  n210 = call <vilib>:"WPI_RobotDriveRefNum Registry Get.vi"("refnum name"="Drivetrain CIM") -> ("RobotDriveDevRef"=w335:T18)  [unwired: 1 in, 9 out]
                  n211 = call-poly <vilib>:"WPI_RobotDriveHolonomicDrive.vi"("Rotation"=0.0, "Y"=-1.0 ("X axis value"), "X"=0.0 ("X axis value"), "RobotDriveDevRef"=w329) -> ("Motor Values"=w330:dbl[])  [unwired: 5 in, 2 out]
                  n212 = call-poly <vilib>:"WPI_RobotDriveHolonomicDrive.vi"("Rotation"=0.0, "Y"=-1.0 ("X axis value"), "X"=0.0 ("X axis value"), "RobotDriveDevRef"=w335) -> ("Motor Values"=w336:dbl[])  [unwired: 5 in, 2 out]
                  n213 = call-poly <vilib>:"NT Write Value.vi"("Numeric Array"=w330) -> ()  [unwired: 10 in, 1 out]
                  n214 = call-poly <vilib>:"NT Write Value.vi"("Numeric Array"=w336) -> ()  [unwired: 10 in, 1 out]
                }
                frame Disabled {
                }
              }
            }
            frame #11 {
              n215 = Wait (ms)(milliseconds to wait=u32 2000) -> ()  [unwired: 1 out]
            }
            frame #12 {
              n216 = disable-structure shown="Enabled" {
                frame Enabled {
                  n217 = call <vilib>:"WPI_RobotDriveRefNum Registry Get.vi"("refnum name"="Drivetrain MiniCIM") -> ("RobotDriveDevRef"=w342:T18)  [unwired: 1 in, 9 out]
                  n218 = call <vilib>:"WPI_RobotDriveRefNum Registry Get.vi"("refnum name"="Drivetrain CIM") -> ("RobotDriveDevRef"=w348:T18)  [unwired: 1 in, 9 out]
                  n219 = call-poly <vilib>:"WPI_RobotDriveHolonomicDrive.vi"("Rotation"=0.0, "Y"=0.0 ("X axis value"), "X"=0.0 ("X axis value"), "RobotDriveDevRef"=w342) -> ("Motor Values"=w343:dbl[])  [unwired: 5 in, 2 out]
                  n220 = call-poly <vilib>:"WPI_RobotDriveHolonomicDrive.vi"("Rotation"=0.0, "Y"=0.0 ("X axis value"), "X"=0.0 ("X axis value"), "RobotDriveDevRef"=w348) -> ("Motor Values"=w349:dbl[])  [unwired: 5 in, 2 out]
                  n221 = call-poly <vilib>:"NT Write Value.vi"("Numeric Array"=w343) -> ()  [unwired: 10 in, 1 out]
                  n222 = call-poly <vilib>:"NT Write Value.vi"("Numeric Array"=w349) -> ()  [unwired: 10 in, 1 out]
                }
                frame Disabled {
                }
              }
            }
            frame #13 {
              n223 = disable-structure shown="Disabled" {
                frame Disabled {
                  n224 = call "2039_hw Brake.vi"() -> ()  [unwired: 2 in, 2 out]
                }
                frame Enabled {
                }
              }
            }
          }
        }
      }
    }
  }
